vi "Gen_TrajLib_Doc_Enum.vi"() -> ()   [LabVIEW 2019]
doc: "Generates and HTML file with the Description of every class, library, ctl, and vi in every open project. Creates separate documents for each library and virtual folder , and links to the top level document. In addition, for every VI shows connector pane. Saves the HTML file in folder <project folder>\\<project name> Documentation\\Documentation.html. erases previous content if any. \nDoes not create documentation for Documentation folder in project if exists. Does not create documentation for packed libraries in the project."
uses:
  Doc_Builder_SubVI/FileAndPath.ctl
  <vilib>/Utility/NIReport.llb/NI_report.lvclass
panel:
  out "Full Library Path":path
  out "Current Section":string
  out "File Index":i32
  out "File Count":i32
  in  "stop":bool
  out "Full Input File Name":path
  in  "GO":bool
  in  "Documentation Path":path=path "../HTML_Build_Work/Temp"
  in  "Library Path":path=path "../../FRC_LV_Trajectory_Library/Enum"
  out "Full Doc Path":path
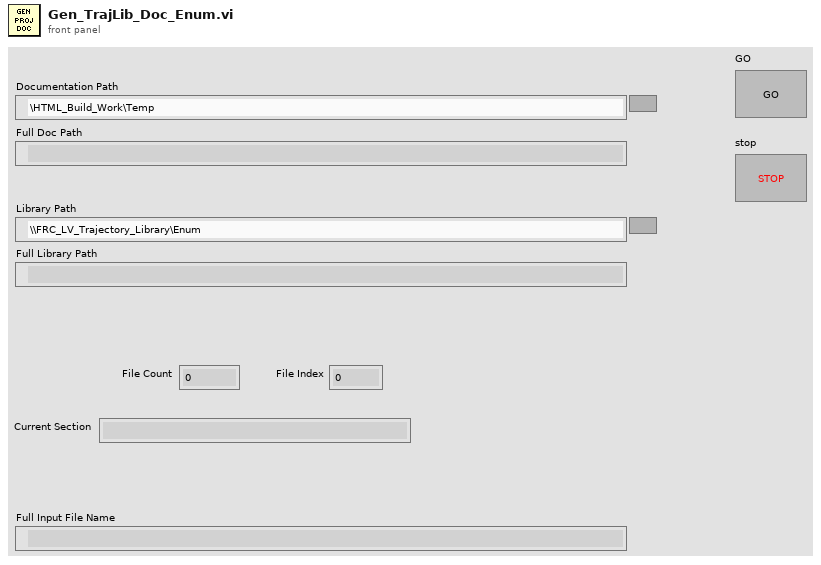
[diagram p1: front panel]
types:
  T1 = typedef "FileAndPath.ctl" = cluster{"FileName":string, "Library Path":path}
  T2 = enum16{"Standard Report", "HTML", "Word", "Excel"}
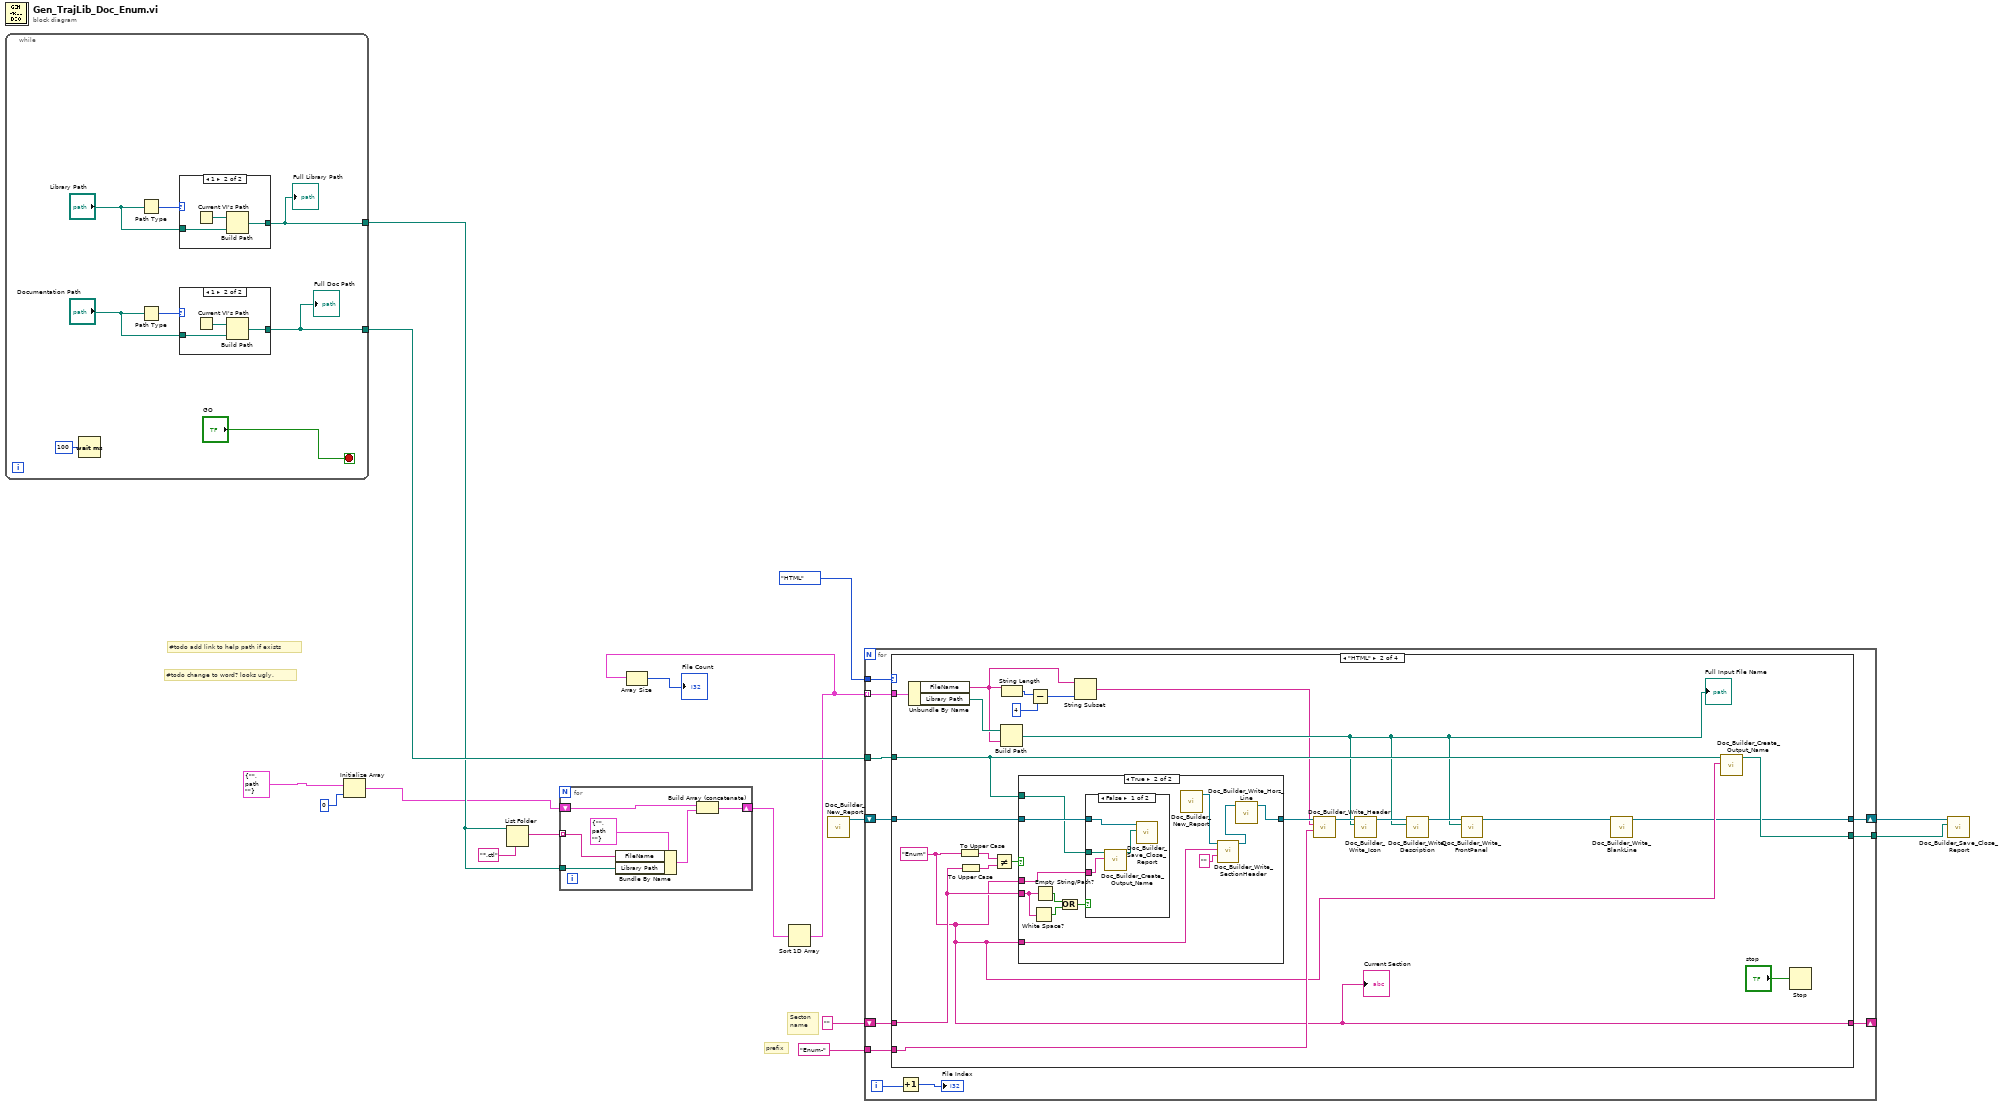
[diagram p0: block diagram]
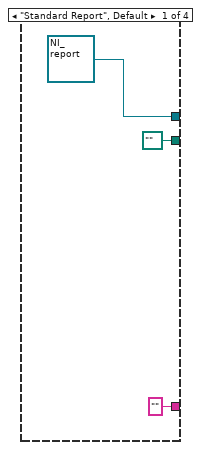
[diagram p4: hidden frame]
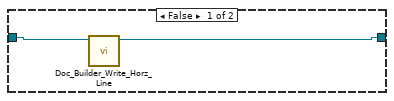
[diagram p5: hidden frame]
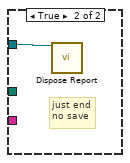
[diagram p6: hidden frame]
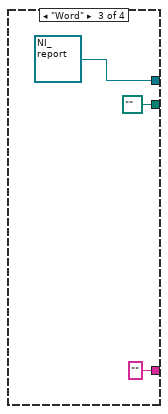
[diagram p7: hidden frame]
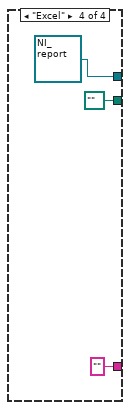
[diagram p8: hidden frame]
diagram:
  # "Secton \nname"
  # "prefix"
  # "#todo change to word? looks ugly."
  # "#todo add link to help path if exists"
  n1 = while {
    tunnel: [w18] -> w14
    tunnel: [w17] -> w10
    stop <- "GO" stop-if-true
    n2 = Wait (ms)(milliseconds to wait=u32 100) -> ()  [unwired: 1 out]
    n3 = Path Type(1:"Library Path") -> (0:w21:i16)
    n4 = Path Type(1:"Documentation Path") -> (0:w22:i16)
    n5 = case shown="1" w21 {
      tunnel: [w25 w27] -> w17
      tunnel: "Library Path" -> [w25 w26]
      frame 0, Default {
      }
      frame 1 {
        n6 = Current VI's Path() -> (path=w28:path)
        n7 = Build Path(base path=w28, name or relative path=w26) -> (appended path=w27:path)
      }
    }
    "Full Library Path" <- w17
    n8 = case shown="1" w22 {
      tunnel: [w29 w31] -> w18
      tunnel: "Documentation Path" -> [w29 w30]
      frame 0, Default {
      }
      frame 1 {
        n9 = Current VI's Path() -> (path=w32:path)
        n10 = Build Path(base path=w32, name or relative path=w30) -> (appended path=w31:path)
      }
    }
    "Full Doc Path" <- w18
  }
  n11 = Initialize Array(T1 {"FileName"="", "Library Path"=path ""} ("FileAndPath"), 0 ("dimension size")) -> (w8:T1[])
  n12 = List Folder(path=w10, pattern="*.ctl") -> (filenames=w11:string[])  [unwired: 2 in, 3 out]
  n13 = for {
    tunnel: w11 -> [w38] mode=indexing
    tunnel: w10 -> [w37]
    shift-right: [w36] -> w1
    shift-left: w8 -> [w35]
    n14 = Bundle By Name(cluster=T1 {"FileName"="", "Library Path"=path ""} ("FileAndPath"), "FileName"=w38, "Library Path"=w37) -> (w33:T1)
    n15 = Build Array (concatenate)(w35, w33) -> (w36:T1[])
  }
  n16 = Sort 1D Array(array=w1) -> (sorted array=w6:T1[])
  n17 = Array Size(array=w6) -> (size(s)=→"File Count":i32)
  n18 = call "Doc_Builder_New_Report.vi"() -> ("NI_report out"=w5:refnum<class "NI_report.lvclass">)  [unwired: 11 in]
  n19 = for {
    tunnel: w6 -> [w48] mode=indexing
    tunnel: T2."HTML" ("report type") -> [w49]
    tunnel: w14 -> [w47]
    tunnel: "Enum-" ("string") -> [w44]
    shift-right: [w40] -> w3
    shift-left: w5 -> [w43]
    shift-right: [w39] -> _
    shift-left: "" ("string") -> [w42]
    tunnel: [w41] -> w2
    i -> [w46]
    n20 = case shown="\"HTML\"" w49 {
      tunnel: w48 -> [_ w70 _ _]
      tunnel: w47 -> [_ w61 _ _]
      tunnel: w44 -> [_ w58 _ _]
      tunnel: w43 -> [_ w65 _ _]
      tunnel: w42 -> [_ w62 _ _]
      tunnel: [path "" ("Full Report Name") w63 path "" ("Full Report Name") path "" ("Full Report Name")] -> w41
      tunnel: [refnum<class "NI_report.lvclass"> refnum ("report out") w53 refnum<class "NI_report.lvclass"> refnum ("report out") refnum<class "NI_report.lvclass"> refnum ("report out")] -> w40
      tunnel: ["" ("FileName") w55 "" ("FileName") "" ("FileName")] -> w39
      frame "Standard Report", Default {
      }
      frame "HTML" {
        w55 = "Enum" ("string")
        n21 = Unbundle By Name(w70) -> ("FileName"=w68:string, "Library Path"=w69:path)
        n22 = To Upper Case(1:w55) -> (0:w67:string)
        n23 = To Upper Case(1:w62) -> (0:w66:string)
        n24 = Not Equal?(x=w67, y=w66) -> (x != y?=w56:bool)
        n25 = Build Path(base path=w69, name or relative path=w68) -> (appended path=w59:path)
        "Full Input File Name" <- w59
        n26 = String Length(string=w68) -> (length=w75:i32)
        n27 = case shown="True" w56 {
          tunnel: w65 -> [w78 w87]
          tunnel: [w77 w84] -> w64
          tunnel: w62 -> [_ w85]
          tunnel: w61 -> [_ w86]
          tunnel: w55 -> [_ w81]
          tunnel: w55 -> [_ w80]
          frame False {
            n28 = call "Doc_Builder_Write_Horz_Line.vi"("NI_report in"=w78) -> ("NI_report out"=w77:refnum<class "NI_report.lvclass">)  [unwired: 10 in]
          }
          frame True {
            n29 = White Space?(1:w85) -> (0:w89:bool)
            n30 = Empty String/Path?(string/path=w85) -> (empty?=w88:bool)
            n31 = Or(x=w88, y=w89) -> (x .or. y?=w90:bool)
            n32 = case shown="False" w90 {
              tunnel: w87 -> [w94 w95]
              tunnel: w86 -> [w93 _]
              tunnel: w80 -> [w92 _]
              frame False {
                n33 = call "Doc_Builder_Create_Output_Name.vi"("Section Name"=w92, "Path"=w93) -> ("Full Report Name"=w91:path)  [unwired: 9 in]
                n34 = call "Doc_Builder_Save_Close_Report.vi"("appended path"=w91, "NI_report in"=w94) -> ()  [unwired: 9 in, 1 out]
              }
              frame True {
                # "just end\nno save"
                n35 = call-dynamic "Dispose Report.vi"("report in"=w95) -> ()  [unwired: 14 in, 1 out]
              }
            }
            n36 = call "Doc_Builder_New_Report.vi"() -> ("NI_report out"=w83:refnum<class "NI_report.lvclass">)  [unwired: 11 in]
            n37 = call "Doc_Builder_Write_SectionHeader.vi"("Prefix String"="", "Section Name"=w81, "NI_report in"=w83) -> ("NI_report out"=w82:refnum<class "NI_report.lvclass">)  [unwired: 8 in]
            n38 = call "Doc_Builder_Write_Horz_Line.vi"("NI_report in"=w82) -> ("NI_report out"=w84:refnum<class "NI_report.lvclass">)  [unwired: 10 in]
          }
        }
        n39 = Subtract(x=w75, y=4) -> (x-y=w73:i32)
        n40 = String Subset(string=w68, length (rest)=w73) -> (substring=w57:string)  [unwired: 1 in]
        n41 = call "Doc_Builder_Write_Header.vi"("Prefix String"=w58, "Item Name"=w57, "NI_report in"=w64) -> ("NI_report out"=w72:refnum<class "NI_report.lvclass">)  [unwired: 8 in]
        n42 = call "Doc_Builder_Write_Icon.vi"("Input Item file path"=w59, "NI_report in"=w72) -> ("NI_report out"=w71:refnum<class "NI_report.lvclass">)  [unwired: 9 in]
        n43 = call "Doc_Builder_Write_Description.vi"("input item file path"=w59, "NI_report in"=w71) -> ("NI_report out"=w60:refnum<class "NI_report.lvclass">)  [unwired: 9 in]
        n44 = call "Doc_Builder_Write_FrontPanel.vi"("input item file path"=w59, "NI_report in"=w60) -> ("NI_report out"=w54:refnum<class "NI_report.lvclass">)  [unwired: 9 in]
        n45 = call "Doc_Builder_Write_BlankLine.vi"("NI_report in"=w54) -> ("NI_report out"=w53:refnum<class "NI_report.lvclass">)  [unwired: 10 in]
        n46 = call "Doc_Builder_Create_Output_Name.vi"("Section Name"=w55, "Path"=w61) -> ("Full Report Name"=w63:path)  [unwired: 9 in]
        n47 = Stop(stop? (T)="stop") -> ()
        "Current Section" <- w55
      }
      frame "Word" {
      }
      frame "Excel" {
      }
    }
    n48 = Increment(x=w46) -> (x+1=→"File Index":i32)
  }
  n49 = call "Doc_Builder_Save_Close_Report.vi"("appended path"=w2, "NI_report in"=w3) -> ()  [unwired: 9 in, 1 out]
